vi "test_Add Response_Variable Number Error.vi"(8 "error in (no error)":errorcluster, 11 "TestCase in":refnum<class "Instrument Addon Scripting API Messages Unit Tests.lvclass">) -> (0 "error out":errorcluster, 3 "TestCase out":refnum<class "Instrument Addon Scripting API Messages Unit Tests.lvclass">)   [LabVIEW 2018, in "Instrument Addon Scripting API Messages Unit Tests.lvclass"]
uses:
  Instrument Addon Scripting API Messages Unit Tests.lvclass
  <vilib>/addons/_JKI Toolkits/VI Tester/TestCase.llb/TestCase.lvclass
  Instrument Addon Scripting API Test Assets/Instrument Addon Scripting API Test Assets.lvclass
  APIs/Scripting API/Instrument Addon Scripting API.lvlib
  <vilib>/NI Veristand/Custom Device API/Custom Device Item Ref.ctl
  <vilib>/NI Veristand/Custom Device API/Custom Device API.lvlib
  APIs/Scripting API/TypeDefs/Linked Channel.ctl
  APIs/Scripting API/TypeDefs/Wait Response Settings.ctl
  APIs/Scripting API/Messages/Add Response - Wait (sec).vi
  <vilib>/NI/NI VeriStand Advanced SysDef API/SysDef API/Advanced System Definition.lvlib
  <vilib>/NI/NI VeriStand Advanced SysDef API/_SubVIs/SysDef.Search.GUID.vi
  Addon/Addon Shared/SubVIs/Constants.vi
  Addon/Addon Shared/Instrument Addon Shared.lvlib
  C:/Program Files (x86)/National Instruments/LabVIEW 2018/vi.lib/addons/_JKI Toolkits/VI Tester/TestCase.llb/TestCase.lvclass
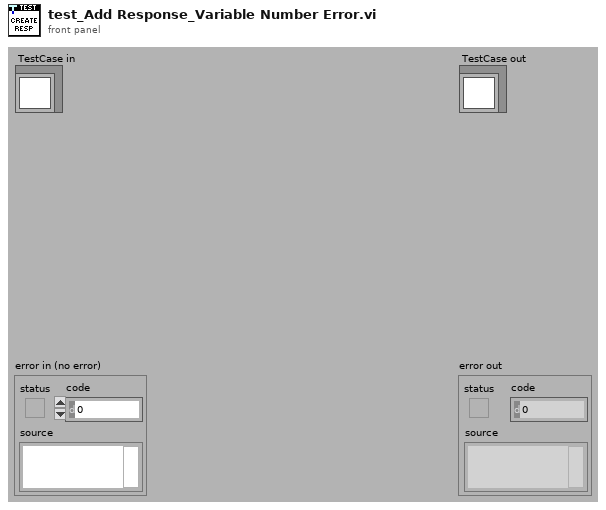
[diagram p1: front panel]
types:
  T1 = typedef "Instrument Addon Scripting API.lvlib/Wait Response Settings.ctl" = cluster{"Response Format":string, "Linked Channels":T2[], "Wait value (sec)":dbl, "Use Wait Channel":bool, "Channel Refnum":T3}
  T2 = typedef "Instrument Addon Scripting API.lvlib/Linked Channel.ctl" = cluster{"Variable Name":string, "Channel Refnum":T3}
  T3 = typedef "Custom Device API.lvlib/Custom Device Item Ref.ctl" = u64
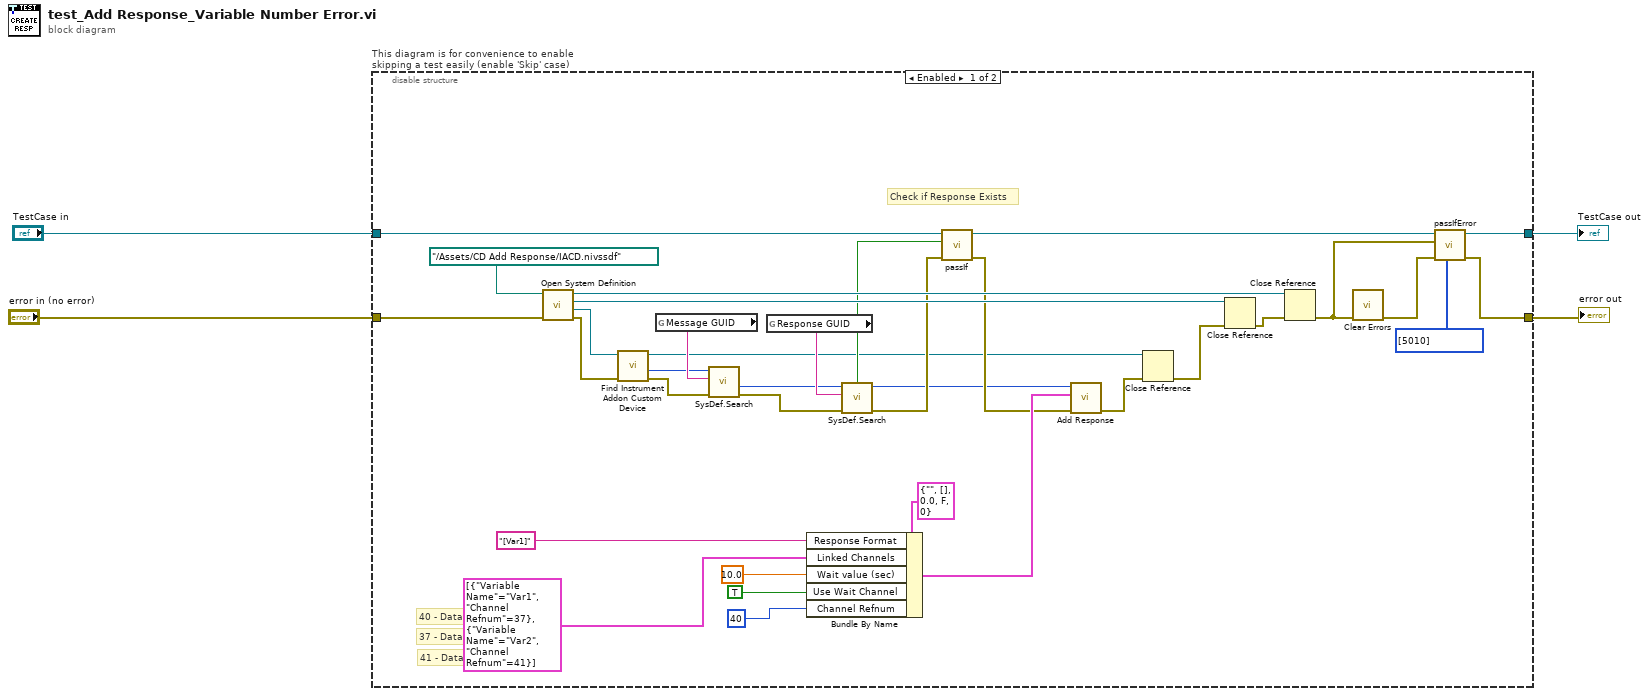
[diagram p0: block diagram]
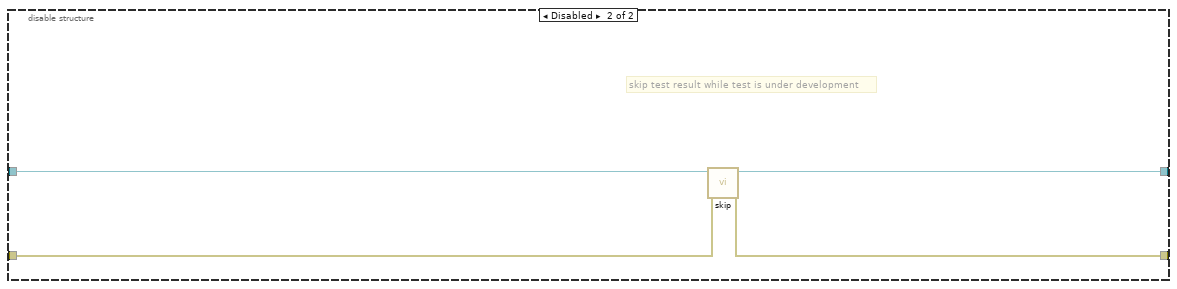
[diagram p2: hidden frame]
diagram:
  n1 = disable-structure "This diagram is for convenience to enable skipping a test easily (enable 'Skip' case)" shown="Enabled" {
    disable-tunnel: "TestCase in" -> [w25 w42]
    disable-tunnel: [w17 w40] -> w1
    disable-tunnel: [w16 w41] -> w3
    disable-tunnel: "error in (no error)" -> [w37 w39]
    frame Enabled {
      # "Check if Response Exists"
      # "41 - Data 2"
      # "40 - Data 0"
      # "37 - Data 1"
      n2 = call "Open System Definition.vi"("error in (no error)"=w37, "System Definition File"=path "../Assets/CD Add Response/IACD.nivssdf" ("SDF file")) -> ("error out"=w35:errorcluster, "Target Refnum"=w34:refnum<k24>, "Root Refnum"=w33:refnum<k24>, "System Definition Refnum"=w28:refnum<k24>)  [unwired: 6 in]
      n3 = call "Find Instrument Addon Custom Device.vi"("error in"=w35, "target in"=w34) -> ("error out"=w11:errorcluster, "NodeID"=w10:u64, "target out"=w6:refnum<k24>)  [unwired: 7 in]
      n4 = global read "Constants.vi" "Message GUID"() -> (w12:string)
      n5 = call-poly <vilib>:"SysDef.Search.vi"("error in (no error)"=w11, "GUID"=w12, "nodeID"=w10) -> ("error out"=w8:errorcluster, "Value out"=w9:u64)  [unwired: 5 in, 2 out]
      n6 = global read "Constants.vi" "Response GUID"() -> (w26:string)
      n7 = Bundle By Name(cluster=T1 {"Response Format"="", "Linked Channels"=[], "Wait value (sec)"=0.0, "Use Wait Channel"=FALSE, "Channel Refnum"=0} ("Settings"), "Response Format"="[Var1]", "Linked Channels"=T2[] [{"Variable Name"="Var1", "Channel Refnum"=37}, {"Variable Name"="Var2", "Channel Refnum"=41}], "Wait value (sec)"=10.0, "Use Wait Channel"=TRUE ("Use Byte Count channel"), "Channel Refnum"=T3 40) -> (w21:T1)
      n8 = call-poly <vilib>:"SysDef.Search.vi"("error in (no error)"=w8, "GUID"=w26, "nodeID"=w9) -> ("error out"=w7:errorcluster, "nodeID out"=w5:u64, "Found?"=w24:bool)  [unwired: 5 in, 1 out]
      n9 = call-dynamic "passIf.vi"("error in (no error)"=w7, "pass"=w24, "TestCase in"=w25) -> ("error out"=w19:errorcluster, "TestCase out"=w18:refnum<class "Instrument Addon Scripting API Messages Unit Tests.lvclass">)  [unwired: 7 in]
      n10 = call-poly "Add Response.vi"("error in (no error)"=w19, "Settings"=w21, "Message in"=w5) -> ("error out"=w20:errorcluster)  [unwired: 7 in, 1 out]
      n11 = Close Reference(reference=w6, error in (no error)=w20) -> (error out=w36:errorcluster)
      n12 = Close Reference(reference=w33, error in (no error)=w36) -> (error out=w27:errorcluster)
      n13 = Close Reference(reference=w28, error in (no error)=w27) -> (error out=w14:errorcluster)
      n14 = call <vilib>:"Clear Errors.vi"("error in (no error)"=w14) -> ("error out"=w13:errorcluster)  [unwired: 5 in, 1 out]
      n15 = call-dynamic "passIfError.vi"("passing error codes (default = any error code)"=i32[] [5010], "error in (no error)"=w13, "error"=w14, "TestCase in"=w18) -> ("error out"=w16:errorcluster, "TestCase out"=w17:refnum<class "Instrument Addon Scripting API Messages Unit Tests.lvclass">)  [unwired: 6 in]
    }
    frame Disabled {
      # "skip test result while test is under development"
      n16 = call <vilib>:"skip.vi"("error in (no error)"=w39, "TestCase in"=w42) -> ("error out"=w41:errorcluster, "TestCase out"=w40:refnum<class "Instrument Addon Scripting API Messages Unit Tests.lvclass">)  [unwired: 8 in]
    }
  }
  "error out" <- w3
  "TestCase out" <- w1
